vi "programa 2.vi"() -> ()   [LabVIEW 2011]
panel:
  out "((A+B)*2)/C":dbl
  in  "C":dbl
  in  "B":dbl
  in  "A":dbl
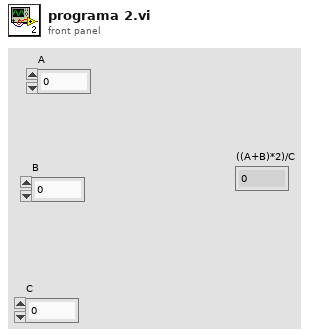
[diagram p1: front panel]
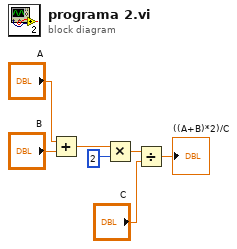
[diagram p0: block diagram]
diagram:
  n1 = Add(x="A", y="B") -> (x+y=w4:dbl)
  n2 = Multiply(x=w4, y=2) -> (x*y=w3:dbl)
  n3 = Divide(x=w3, y="C") -> (x/y=→"((A+B)*2)/C":dbl)
